vi "UNIX to LabVIEW.vi"(1 "UNIX Time":i32) -> (0 "LabVIEW Time":dbl)   [LabVIEW 2009]
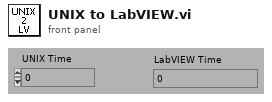
[diagram p1: front panel]
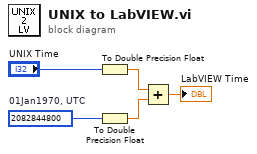
[diagram p0: block diagram]
diagram:
  w5 = 2082844800  # 01Jan1970, UTC
  n1 = To Double Precision Float(number="UNIX Time") -> (double precision float=w2:dbl)
  n2 = To Double Precision Float(number=w5) -> (double precision float=w1:dbl)
  n3 = Add(x=w2, y=w1) -> (x+y=→"LabVIEW Time":dbl)
